vi "启动参数显隐控制.vi"(0 "启动参数":refnum<vi>, 3 "error in (no error)":errorcluster) -> (10 "error out":errorcluster)   [LabVIEW 2016]
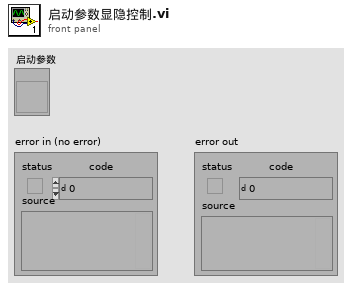
[diagram p1: front panel]
types:
  T1 = typedef "启动参数.ctl" = cluster{"氨氮":bool, "总磷":bool, "总氮":bool, "多参数":bool, "CODmn":bool, "CODCr":bool, "氟化物":bool, "超标留样":bool, "重金属":bool, "挥发酚":bool, "综合生物毒性":bool}
  T2 = typedef "模块配置类型.ctl" = enum16{"单模块", "总磷总氮二合一模块", "氨氮总磷二合一模块"}
  T3 = typedef "氨氮总磷总氮模块版本.ctl" = enum16{"V2", "V3"}
  T4 = cluster{"[0]":bool, "[1]":bool, "[2]":bool, "[3]":bool, "[4]":bool, "[5]":bool, "[6]":bool, "[7]":bool, "[8]":bool, "[9]":bool, "[10]":bool}
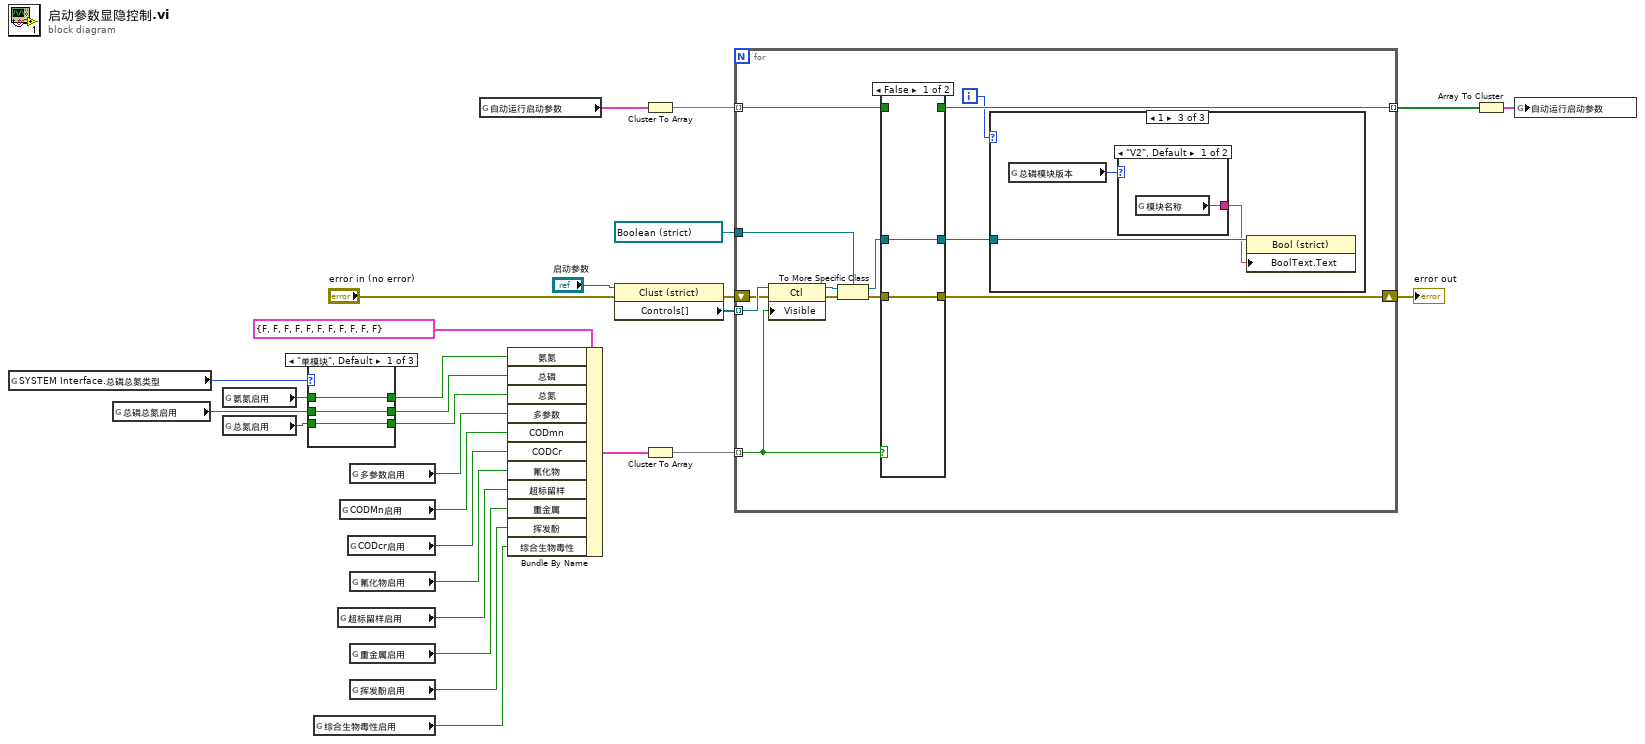
[diagram p0: block diagram]
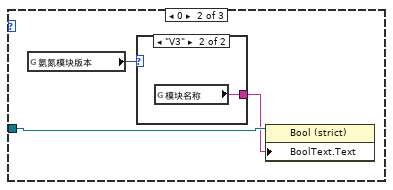
[diagram p5: hidden frame]
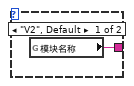
[diagram p6: hidden frame]
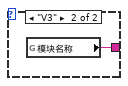
[diagram p7: hidden frame]
diagram:
  n1 = global read "系统设置全局变量.vi" "SYSTEM Interface.总磷总氮类型"() -> (w13:T2)
  n2 = global read "系统设置全局变量.vi" "总磷总氮启用"() -> (w10:bool)
  n3 = global read "系统设置全局变量.vi" "氨氮启用"() -> (w12:bool)
  n4 = global read "系统设置全局变量.vi" "总氮启用"() -> (w11:bool)
  n5 = case shown="\"单模块\", Default" w13 {
    tunnel: [w29 w33 w35] -> w9
    tunnel: [w30 w33 w34] -> w8
    tunnel: [w31 w32 w35] -> w7
    tunnel: w12 -> [w31 w32 w35]
    tunnel: w11 -> [w30 _ w34]
    tunnel: w10 -> [w29 w33 _]
    frame "单模块", Default {
    }
    frame "总磷总氮二合一模块" {
    }
    frame "氨氮总磷二合一模块" {
    }
  }
  n6 = global read "系统设置全局变量.vi" "综合生物毒性启用"() -> (w2:bool)
  n7 = global read "系统设置全局变量.vi" "超标留样启用"() -> (w23:bool)
  n8 = global read "系统设置全局变量.vi" "CODMn启用"() -> (w21:bool)
  n9 = global read "系统设置全局变量.vi" "CODcr启用"() -> (w18:bool)
  n10 = global read "系统设置全局变量.vi" "多参数启用"() -> (w20:bool)
  n11 = global read "系统设置全局变量.vi" "氟化物启用"() -> (w22:bool)
  n12 = global read "系统设置全局变量.vi" "重金属启用"() -> (w19:bool)
  n13 = global read "系统设置全局变量.vi" "挥发酚启用"() -> (w17:bool)
  n14 = global read "系统设置全局变量.vi" "自动运行启动参数"() -> (w6:T1)
  n15 = Bundle By Name(cluster=T1 {"氨氮"=FALSE, "总磷"=FALSE, "总氮"=FALSE, "多参数"=FALSE, "CODmn"=FALSE, "CODCr"=FALSE, "氟化物"=FALSE, "超标留样"=FALSE, "重金属"=FALSE, "挥发酚"=FALSE, "综合生物毒性"=FALSE} ("显隐设置"), "氨氮"=w7, "总磷"=w9, "总氮"=w8, "多参数"=w20, "CODmn"=w21, "CODCr"=w18, "氟化物"=w22, "超标留样"=w23, "重金属"=w19, "挥发酚"=w17, "综合生物毒性"=w2) -> (w24:T1)
  n16 = property class="Clust (strict)"(reference="启动参数", error in="error in (no error)") -> (error out=w16:errorcluster, "Controls[]"=w25:refnum<vi>[])  [unwired: 1 out]
  n17 = Cluster To Array(cluster=w6) -> (array=w5:bool[])
  n18 = Cluster To Array(cluster=w24) -> (array=w27:bool[])
  n19 = for {
    tunnel: w25 -> [w48] mode=indexing
    tunnel: w27 -> [w43] mode=indexing
    tunnel: refnum<vi> refnum ("氨氮") -> [w45]
    shift-right: [w38] -> w15
    shift-left: w16 -> [w42]
    tunnel: w5 -> [w40] mode=indexing
    tunnel: [w39] -> w4 mode=indexing
    i -> [w36]
    n20 = property class="Ctl"(reference=w48, error in=w42, "Visible"=w43) -> (reference out=w47:refnum<vi>, error out=w46:errorcluster)
    n21 = To More Specific Class(target class=w45, reference=w47, error in=w46) -> (specific class reference=w44:refnum<vi>, error out=w41:errorcluster)
    n22 = case shown="False" w43 {
      tunnel: w44 -> [w60 w63]
      tunnel: [w60 w63] -> w37
      tunnel: [w59 w62] -> w38
      tunnel: w41 -> [w59 w62]
      tunnel: w40 -> [_ w61]
      tunnel: [_ w61] -> w39
      frame False {
      }
      frame True {
      }
    }
    n23 = case shown="1" w36 {
      tunnel: w37 -> [_ w51 w56]
      frame Default {
      }
      frame 0 {
        n24 = global read "系统设置全局变量.vi" "氨氮模块版本"() -> (w50:T3)
        n25 = case shown="\"V3\"" w50 {
          tunnel: [w52 w53] -> w49
          frame "V2", Default {
            n26 = global read "VAR总磷总氮全局变量.vi" "模块名称"() -> (w52:string)
          }
          frame "V3" {
            n27 = global read "VAR总磷总氮全局变量.vi" "模块名称"() -> (w53:string)
          }
        }
        n28 = property class="Bool (strict)"(reference=w51, "BoolText.Text"=w49) -> ()  [unwired: 1 in, 2 out]
      }
      frame 1 {
        n29 = global read "系统设置全局变量.vi" "总磷模块版本"() -> (w55:T3)
        n30 = case shown="\"V2\", Default" w55 {
          tunnel: [w57 w58] -> w54
          frame "V2", Default {
            n31 = global read "VAR总磷总氮全局变量.vi" "模块名称"() -> (w57:string)
          }
          frame "V3" {
            n32 = global read "VAR总磷总氮全局变量.vi" "模块名称"() -> (w58:string)
          }
        }
        n33 = property class="Bool (strict)"(reference=w56, "BoolText.Text"=w54) -> ()  [unwired: 1 in, 2 out]
      }
    }
  }
  "error out" <- w15
  n34 = Array To Cluster(array=w4) -> (cluster=w3:T4)
  n35 = global write "系统设置全局变量.vi" "自动运行启动参数"(w3) -> ()
